vi "Scripting_PlaceGoopRefInClassAttribute.vi"(4 "error in":errorcluster, 6 "ObjectRef_LvClassFolderPath":path, 7 "ClassRefnum":refnum<vi>) -> (0 "error out":errorcluster, 1 "ClusterTypeDefPath":path, 2 "ObjectRef.ctl":path, 3 "ReplacedObjectRef(ifOldRefFound)":path)   [LabVIEW 2020]
uses:
  <vilib>/Utility/miscctls.llb/LVPointTypeDef.ctl
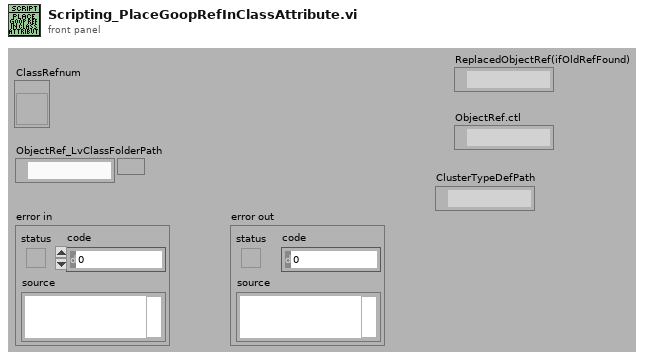
[diagram p1: front panel]
types:
  T1 = typedef "LVPointTypeDef.ctl" = cluster{"Horizontal":i16, "Vertical":i16}
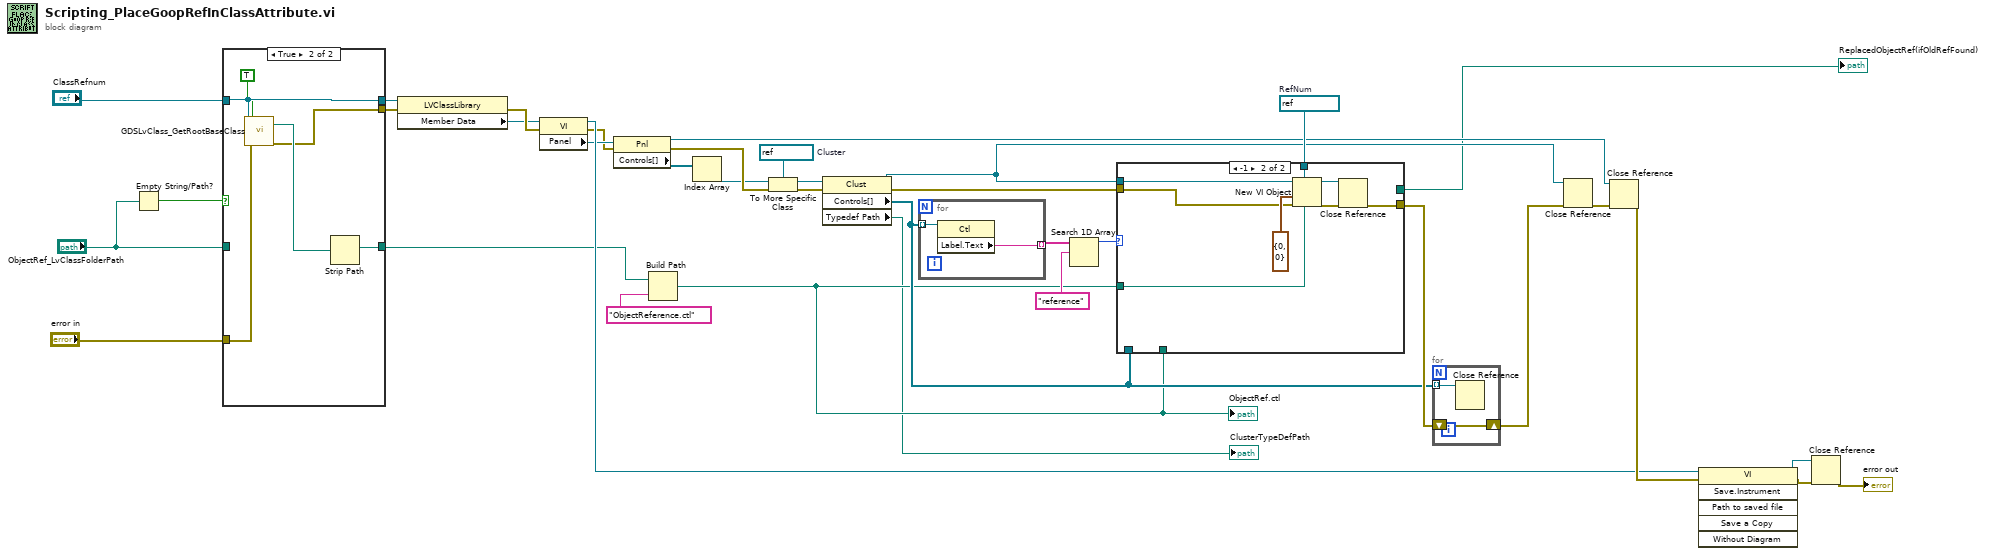
[diagram p0: block diagram]
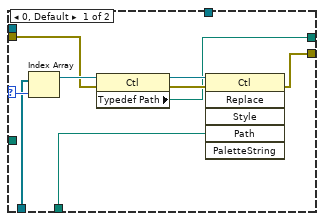
[diagram p3: hidden frame]
diagram:
  w34 = refnum<vi> refnum  # RefNum
  w26 = refnum<vi> refnum  # Cluster
  n1 = Empty String/Path?(string/path="ObjectRef_LvClassFolderPath") -> (empty?=w9:bool)
  n2 = case shown="True" w9 {
    tunnel: "ObjectRef_LvClassFolderPath" -> [w40 _]
    tunnel: [w40 w46] -> w7
    tunnel: "ClassRefnum" -> [w39 w44]
    tunnel: [w39 w44] -> w5
    tunnel: "error in" -> [w38 w45]
    tunnel: [w38 w42] -> w3
    frame False {
    }
    frame True {
      n3 = call <resource>:"GDSLvClass_GetRootBaseClass.vi"("ViRef/Path,LvClassRef/Path"=w44, "error in (no error)"=w45, "Don'tOpenReference"=TRUE) -> ("RootBaseClassPath"=w43:path, "error out"=w42:errorcluster)  [unwired: 11 in, 4 out]
      n4 = Strip Path(path=w43) -> (stripped path=w46:path)  [unwired: 1 out]
    }
  }
  n5 = property class="LVClassLibrary"(reference=w5, error in=w3) -> (error out=w23:errorcluster, "Member Data"=w21:refnum<vi>)  [unwired: 1 out]
  n6 = property class="VI"(reference=w21, error in=w23) -> (reference out=w36:refnum<vi>, error out=w22:errorcluster, "Panel"=w24:refnum<vi>)
  n7 = property class="Pnl"(reference=w24, error in=w22) -> (reference out=w30:refnum<vi>, error out=w28:errorcluster, "Controls[]"=w25:refnum<vi>[])
  n8 = Build Path(base path=w7, name or relative path="ObjectReference.ctl") -> (appended path=w2:path)
  "ObjectRef.ctl" <- w2
  n9 = Index Array(array=w25) -> (element=w27:refnum<vi>)  [unwired: 1 in]
  n10 = To More Specific Class(target class=w26, reference=w27, error in=w28) -> (specific class reference=w20:refnum<vi>, error out=w19:errorcluster)
  n11 = property class="Clust"(reference=w20, error in=w19) -> (reference out=w18:refnum<vi>, error out=w14:errorcluster, "Controls[]"=w11:refnum<vi>[], "Typedef Path"=→"ClusterTypeDefPath":path)
  n12 = for {
    tunnel: w11 -> [w48] mode=indexing
    tunnel: [w47] -> w17 mode=indexing
    n13 = property class="Ctl"(reference=w48) -> ("Label.Text"=w47:string)  [unwired: 1 in, 2 out]
  }
  n14 = Search 1D Array(1D array=w17, element="reference") -> (index of element=w15:i32)  [unwired: 1 in]
  n15 = case shown="-1" w15 {
    selector: w15 -> [w57 _]
    tunnel: w34 -> [_ w65]
    tunnel: [w54 w63] -> w12
    tunnel: w2 -> [_ w60]
    tunnel: w18 -> [_ w59]
    tunnel: w14 -> [w52 w58]
    tunnel: w11 -> [w56 _]
    tunnel: w2 -> [w55 _]
    tunnel: [w49 _] -> w10
    frame 0, Default {
      n16 = Index Array(array=w56, index=w57) -> (element=w53:refnum<vi>)
      n17 = property class="Ctl"(reference=w53, error in=w52) -> (reference out=w51:refnum<vi>, error out=w50:errorcluster, "Typedef Path"=w49:path)
      n18 = invoke class="Ctl" method="Replace"(reference=w51, error in=w50, "Path"=w55) -> (error out=w54:errorcluster)  [unwired: 3 in, 5 out]
    }
    frame -1 {
      n19 = New VI Object(vi object class=w65, owner refnum=w59, position/next to=T1 {"Horizontal"=0, "Vertical"=0} ("relative position/next to refnum"), 6:w60, 8:w58) -> (object refnum=w62:refnum<vi>, 0:w61:errorcluster)  [unwired: 3 in]
      n20 = Close Reference(reference=w62, error in (no error)=w61) -> (error out=w63:errorcluster)
    }
  }
  "ReplacedObjectRef(ifOldRefFound)" <- w10
  n21 = for {
    shift-right: [w66] -> w13
    shift-left: w12 -> [w66]
    tunnel: w11 -> [w67] mode=indexing
    n22 = Close Reference(reference=w67) -> ()  [unwired: 1 in, 1 out]
  }
  n23 = Close Reference(reference=w18, error in (no error)=w13) -> (error out=w29:errorcluster)
  n24 = Close Reference(reference=w30, error in (no error)=w29) -> (error out=w37:errorcluster)
  n25 = invoke class="VI" method="Save.Instrument"(reference=w36, error in=w37) -> (reference out=w32:refnum<vi>, error out=w31:errorcluster)  [unwired: 4 in, 4 out]
  n26 = Close Reference(reference=w32, error in (no error)=w31) -> (error out=→"error out":errorcluster)
